vi "o3 Serial Data Driver.vi"() -> ()   [LabVIEW 2010]
uses:
  <vilib>/Instr/_visa.llb/VISA Set IO Buffer Mask.ctl
  <vilib>/Platform/TimedLoop/XDataNode/XDataNode.xnode
  <vilib>/Platform/TimedLoop/XDataNode/timing_clust.ctl
  <vilib>/Platform/TimedLoop/XDataNode/nitl_modes.ctl
  <vilib>/Platform/TimedLoop/XDataNode/wakeup.ctl
  <vilib>/Instr/_visa.llb/VISA Configure Serial Port (Instr).vi
  <vilib>/Platform/TimedLoop/XDataNode/XDNodeRunTimeDep.lvlib
panel:
  in  "milliseconds to wait":u32
  in  "timeout (10sec)":u32=500
  out "Array":string[](array[string])
  in  "Byte":u32[](array[numeric])
  in  "Command":string[](array[string])
  out "Waveform Chart":u32(graph)
  in  "ID":string="±"
  in  "VISA resource name":refnum<visa-resource-name>="COM1"
  out "Number of times \nRead time out":u32
  out "Max Time diff":u32
  out "Time diff":u32
  out "Loop count":i32
  out "concatenated string":string
  out "error out":errorcluster
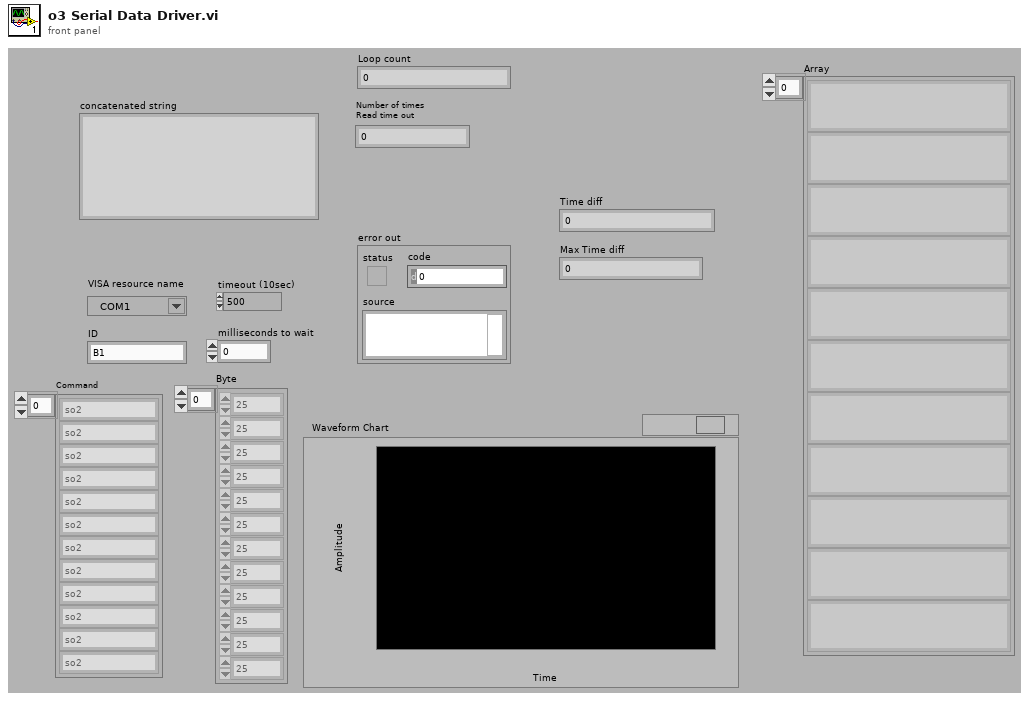
[diagram p1: front panel]
types:
  T1 = typedef "XDNodeRunTimeDep.lvlib/timing_clust.ctl" = cluster{"Expected End [f-1]":u64, "Actual End [f-1]":u64, "Finished Late? [f-1]":bool, "Expected End [i-1]":u64, "Actual End [i-1]":u64, "Finished Late? [i-1]":bool, "Expected Start [i]":u64, "Actual Start [i]":u64, "Expected Start [f]":u64, "Actual Start [f]":u64, "Source Name":string, "Structure Name":string, "Period":i64, "Deadline":i64, "Offset":i64, "Start":i64, "Priority":i32, "Timeout":i32, "Mode":T2, "Wakeup Reason":T3, "Error":errorcluster, "Source Type":string, "Secondary Source Type":string, "Global End Time":u64, "Global Start Time":u64, "Frame Duration":u64, "Iteration Duration":u64, "Assigned CPU":i32, "I/O Scan Engine Mode":u32}
  T2 = typedef "XDNodeRunTimeDep.lvlib/nitl_modes.ctl" = enum32{"No Change", "Process missed periods, maintain original phase", "Discard missed periods, maintain original phase", "Process missed periods, ignore original phase", "Discard missed periods, ignore original phase"}
  T3 = typedef "XDNodeRunTimeDep.lvlib/wakeup.ctl" = enum32{"Normal", "Aborted", "Asynchronous wakeup", "Timing source error", "Timed loop error", "Timeout"}
  T4 = typedef "VISA Set IO Buffer Mask.ctl" = u16
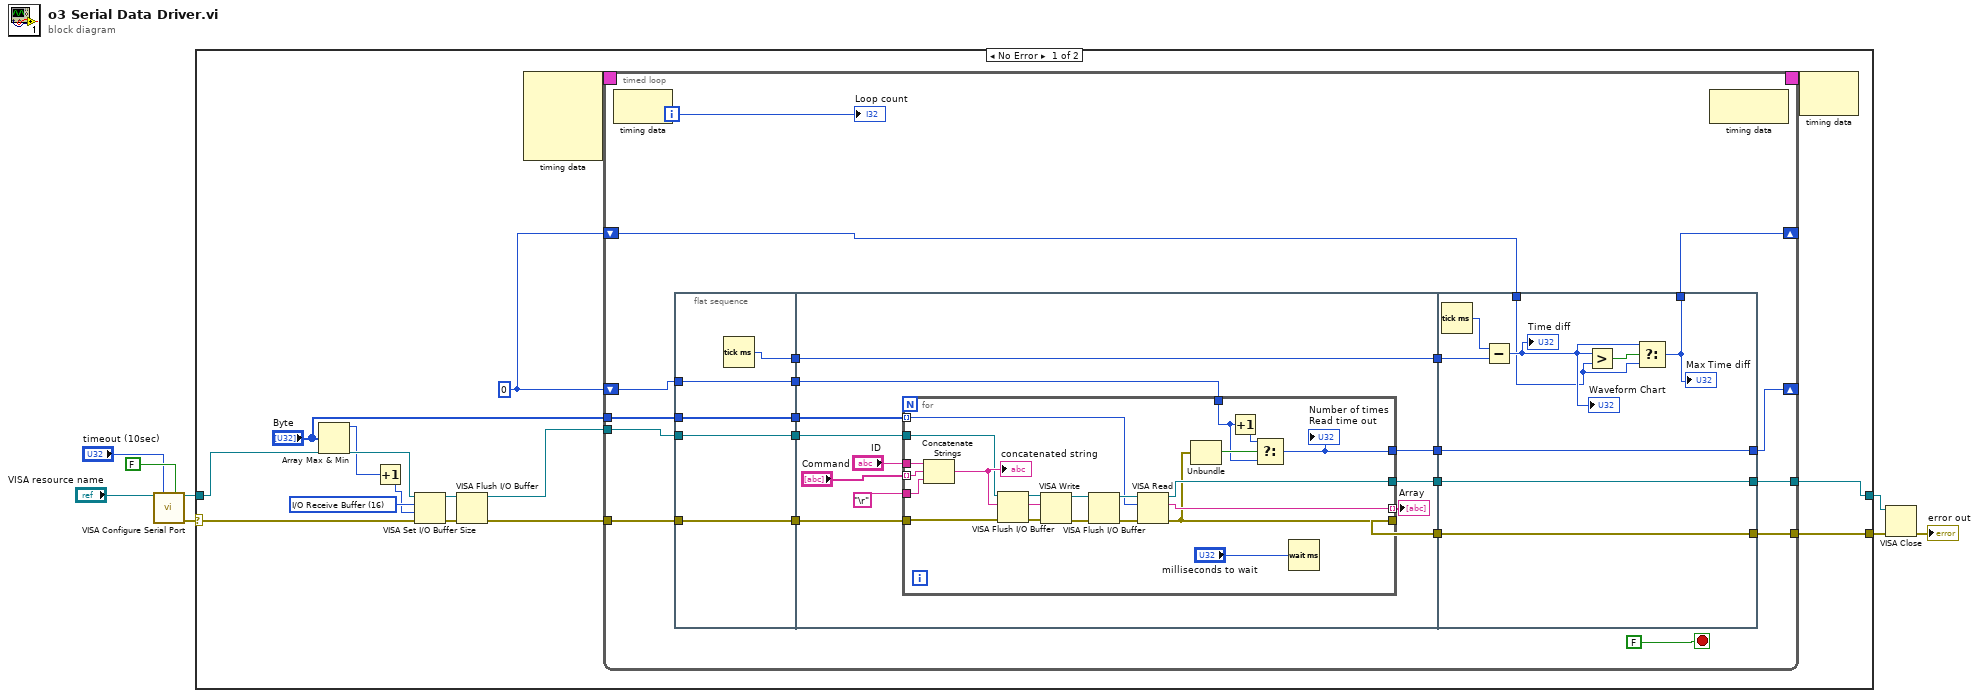
[diagram p0: block diagram]
diagram:
  n1 = call-poly "VISA Configure Serial Port"("VISA resource name"="VISA resource name", "timeout (10sec)"="timeout (10sec)", "Enable Termination\nChar (T)"=FALSE ("Enable Termination\nChar (T)")) -> ("VISA resource name out"=w8:refnum<visa-resource-name>, "error out"=w3:errorcluster)  [unwired: 11 in]
  n2 = case shown="No Error" w3 {
    selector: w3 -> [w19 w95]
    tunnel: w8 -> [w20 w96]
    tunnel: [w15 w96] -> w6
    tunnel: [w21 w95] -> w5
    frame No Error {
      w16 = T4 16 items=["I/O Receive Buffer"=16, "I/O Transmit Buffer"=32, "I/O Receive and Transmit Buffer"=48] ("Mask")
      w14 = u32 0
      n3 = Array Max & Min(array="Byte") -> (max value=w12:u32)  [unwired: 3 out]
      n4 = Increment(x=w12) -> (x+1=w11:u32)
      n5 = VISA Set I/O Buffer Size(VISA resource name=w20, mask (16)=w16, size (4096)=w11, error in (no error)=w19) -> (VISA resource name out=w17:refnum<visa-resource-name>, error out=w18:errorcluster)
      n6 = VISA Flush I/O Buffer(VISA resource name=w17, error in (no error)=w18) -> (VISA resource name out=w23:refnum<visa-resource-name>, error out=w22:errorcluster)  [unwired: 1 in]
      n7 = node-c288() -> (w10:T1)  [unwired: 4 in]
      n8 = timed-loop {
        tunnel: w23 -> [w43]
        tunnel: w22 -> [w42]
        tunnel: [w40] -> w21
        shift-right: [w35] -> _
        shift-left: w14 -> [w36]
        shift-right: [w24] -> _
        shift-left: w14 -> [w25]
        tunnel: [w39] -> w15
        tunnel: "Byte" -> [w37]
        timing: w10 -> [_]
        timing-out: [_] -> w9
        i -> [w38]
        stop <- FALSE stop-if-true
        n9 = node-c288() -> ()  [unwired: 1 in, 1 out]
        n10 = flat-sequence {
          tunnel: w36 -> [w47]
          tunnel: w37 -> [w48]
          tunnel: w42 -> [w49]
          tunnel: w43 -> [w50]
          tunnel: [w50] -> w34
          tunnel: [w49] -> w33
          tunnel: [w48] -> w32
          tunnel: [w47] -> w31
          tunnel: [w46] -> w26
          tunnel: w34 -> [w62]
          tunnel: w33 -> [w61]
          tunnel: w32 -> [w55]
          tunnel: w31 -> [w54]
          tunnel: [w60] -> w30
          tunnel: [w59] -> w29
          tunnel: [w53] -> w28
          tunnel: [w51] -> w27
          tunnel: w26 -> [w51]
          tunnel: [w90] -> w35
          tunnel: [w91] -> w39
          tunnel: [w92] -> w40
          tunnel: w30 -> [w92]
          tunnel: w29 -> [w91]
          tunnel: w28 -> [w90]
          tunnel: w27 -> [w86]
          tunnel: w25 -> [w85]
          tunnel: [w84] -> w24
          frame #0 {
            n11 = Tick Count (ms)() -> (millisecond timer value=w46:u32)
          }
          frame #1 {
            n12 = for {
              tunnel: w62 -> [w67]
              tunnel: w61 -> [w64]
              tunnel: [w72] -> w60
              tunnel: [w82] -> w59
              tunnel: "\r" -> [w80]
              tunnel: "ID" -> [w78]
              tunnel: [w77] -> w52 mode=indexing
              tunnel: "Command" -> [w74] mode=indexing
              tunnel: w55 -> [w73] mode=indexing
              tunnel: w54 -> [w69]
              tunnel: [w68] -> w53
              n13 = Concatenate Strings(w78, w74, w80) -> (w79:string)
              "concatenated string" <- w79
              n14 = VISA Flush I/O Buffer(VISA resource name=w67, error in (no error)=w64) -> (VISA resource name out=w66:refnum<visa-resource-name>, error out=w65:errorcluster)  [unwired: 1 in]
              n15 = VISA Write(VISA resource name=w66, write buffer=w79, error in (no error)=w65) -> (VISA resource name out=w81:refnum<visa-resource-name>, error out=w83:errorcluster)  [unwired: 1 out]
              n16 = VISA Flush I/O Buffer(VISA resource name=w81, error in (no error)=w83) -> (VISA resource name out=w76:refnum<visa-resource-name>, error out=w75:errorcluster)  [unwired: 1 in]
              n17 = VISA Read(VISA resource name=w76, byte count=w73, error in (no error)=w75) -> (VISA resource name out=w82:refnum<visa-resource-name>, read buffer=w77:string, error out=w72:errorcluster)  [unwired: 1 out]
              n18 = Unbundle(w72) -> ("status"=w71:bool)  [unwired: 2 out]
              n19 = Increment(x=w69) -> (x+1=w70:u32)
              n20 = Select(t=w70, s=w71, f=w69) -> (s? t:f=w68:u32)
              "Number of times \nRead time out" <- w68
              n21 = Wait (ms)(milliseconds to wait="milliseconds to wait") -> ()  [unwired: 1 out]
            }
            "Array" <- w52
          }
          frame #2 {
            n22 = Tick Count (ms)() -> (millisecond timer value=w89:u32)
            n23 = Subtract(x=w89, y=w86) -> (x-y=w88:u32)
            "Time diff" <- w88
            "Waveform Chart" <- w88
            n24 = Greater?(x=w88, y=w85) -> (0:w87:bool)
            n25 = Select(t=w88, s=w87, f=w85) -> (s? t:f=w84:u32)
            "Max Time diff" <- w84
          }
        }
        n26 = node-c288() -> ()  [unwired: 1 in, 1 out]
        "Loop count" <- w38
      }
      n27 = node-c288(w9) -> ()  [unwired: 1 out]
    }
    frame Error {
    }
  }
  n28 = VISA Close(VISA resource name=w6, error in (no error)=w5) -> (error out=→"error out":errorcluster)
